vi "Beam Breaker.vi"(0 "Mode":enum8{"Start", "Run", "Finish"}(ring)) -> (1 "Clamp Wide":bool)   [LabVIEW 2014]
uses:
  <vilib>/Rock Robotics/SystemInterfaces/DIO/FPGA_DIOChannel.ctl
  <vilib>/Rock Robotics/Network Tables/SD Write Boolean.vi
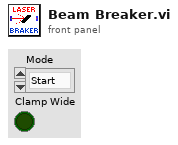
[diagram p1: front panel]
types:
  T1 = typedef "FPGA_DIOChannel.ctl" = enum8{"DIO 0", "DIO 1", "DIO 2", "DIO 3", "DIO 4", "DIO 5", "DIO 6", "DIO 7", "DIO 8", "DIO 9", "DIO MXP 0", "DIO MXP 1", "DIO MXP 2", "DIO MXP 3", "DIO MXP 4", "DIO MXP 5", "DIO MXP 6", "DIO MXP 7", "DIO MXP 8", "DIO MXP 9", "DIO MXP 10", "DIO MXP 11", "DIO MXP 12", "DIO MXP 13", "DIO MXP 14", "DIO MXP 15", "Invalid"}
  T2 = typedef "WPI_DigitalInputDevRef.ctl" = cluster{"DevStatus":errorcluster, "DIO Channel":T1, "Controller":T3}
  T3 = typedef "FPGA_TypedefDigitalModule.ctl" = enum16{"Controller 1"}
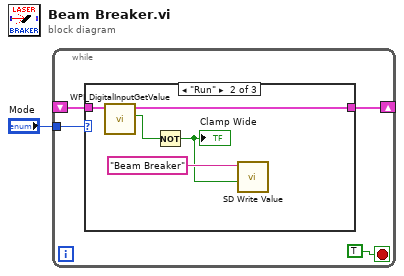
[diagram p0: block diagram]
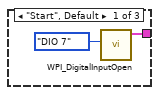
[diagram p2: hidden frame]
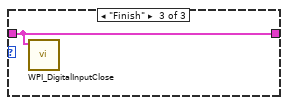
[diagram p3: hidden frame]
diagram:
  n1 = while {
    tunnel: "Mode" -> [w5]
    shift-right: [w4] -> _
    shift-left: _ -> [w3]
    stop <- TRUE stop-if-true
    n2 = case shown="\"Run\"" w5 {
      tunnel: [w6 w11 w13] -> w4
      tunnel: w3 -> [_ w12 w13]
      frame "Start", Default {
        n3 = call <vilib>:"WPI_DigitalInputOpen.vi"("DIO Channel"=FPGA_DIOChannel."DIO 7") -> ("DigitalInputDevRef"=w6:T2)  [unwired: 9 in, 1 out]
      }
      frame "Run" {
        n4 = call <vilib>:"WPI_DigitalInputGetValue.vi"("DigitalInputDevRef"=w12) -> ("Value"=w9:bool, "DigitalInputDevRef"=w11:T2)  [unwired: 8 in, 1 out]
        n5 = Not(x=w9) -> (.not. x?=w8:bool)
        "Clamp Wide" <- w8
        n6 = call-poly <vilib>:"SD Write Value.vi"("Boolean"=w8, "Name"="Beam Breaker") -> ()  [unwired: 8 in, 2 out]
      }
      frame "Finish" {
        n7 = call <vilib>:"WPI_DigitalInputClose.vi"("DigitalInputDevRef"=w13) -> ()  [unwired: 10 in, 1 out]
      }
    }
  }
